vi "Update Mouse Move.vi"(8 "error in (no error)":errorcluster, 10 "Mouse Move":T1, 11 "Map Model in":refnum<class "Map Model.lvclass">) -> (0 "error out":errorcluster, 3 "Map Model out":refnum<class "Map Model.lvclass">)   [LabVIEW 2020, in "Map Model.lvlib" / "Map Model.lvclass"]
uses:
  Map Model.lvclass
  <vilib>/Utility/miscctls.llb/LVPoint32TypeDef.ctl
  Map Model.lvclass/Map Model.ctl
  Tools/Tool/Tool.lvclass
panel:
  # "NOTICE -- YOU MUST LEAVE THIS NOTICE IN PLACE.\n\nCopyright (c) 2017, LIANG LIU Shawn.Liu.cn@gmail.com\nAll rights reserved.\n\nRedistribution and use in source and binary forms, with or without modification, are permitted provided that the following conditions are met:\n-Redistributions of source code must retain the above copyright notice, this list of conditions and the following disclaimer.\n-Redistributions in binary form must reproduce the above copyright notice, this list of conditions and the following disclaimer in the documentation and/or other materials provided with the distribution.\n-Neither the name of the eLp nor the names of its contributors may be used to endorse or promote products derived from this software without specific prior written permission.\n\nTHIS SOFTWARE IS PROVIDED BY THE COPYRIGHT HOLDERS AND CONTRIBUTORS \"AS IS\" AND ANY EXPRESS OR IMPLIED WARRANTIES, INCLUDING, BUT NOT LIMITED TO, THE IMPLIED WARRANTIES OF MERCHANTABILITY AND FITNESS FOR A PARTICULAR PURPOSE ARE DISCLAIMED. IN NO EVENT SHALL THE COPYRIGHT HOLDER OR CONTRIBUTORS BE LIABLE FOR ANY DIRECT, INDIRECT, INCIDENTAL, SPECIAL, EXEMPLARY, OR CONSEQUENTIAL DAMAGES (INCLUDING, BUT NOT LIMITED TO, PROCUREMENT OF SUBSTITUTE GOODS OR SERVICES; LOSS OF USE, DATA, OR PROFITS; OR BUSINESS INTERRUPTION) HOWEVER CAUSED AND ON ANY THEORY OF LIABILITY, WHETHER IN CONTRACT, STRICT LIABILITY, OR TORT (INCLUDING NEGLIGENCE OR OTHERWISE) ARISING IN ANY WAY OUT OF THE USE OF THIS SOFTWARE, EVEN IF ADVISED OF THE POSSIBILITY OF SUCH DAMAGE."
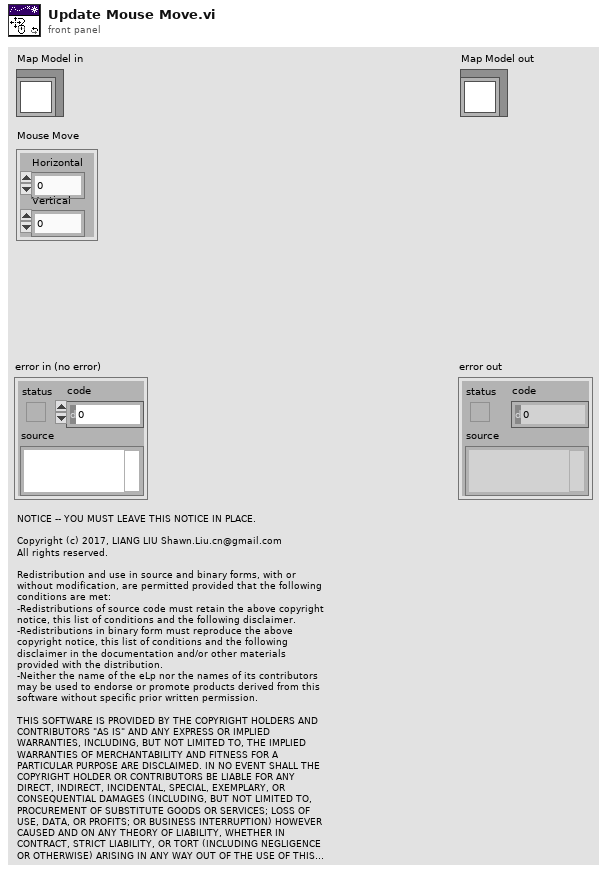
[diagram p1: front panel]
types:
  T1 = typedef "LVPoint32TypeDef.ctl" = cluster{"Horizontal":i32, "Vertical":i32}
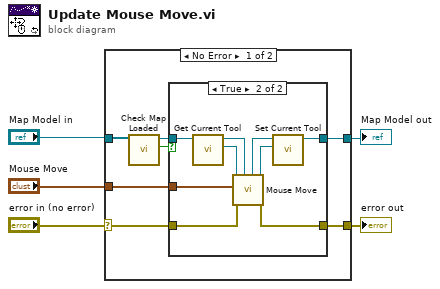
[diagram p0: block diagram]
diagram:
  n1 = case shown="No Error" "error in (no error)" {
    selector: "error in (no error)" -> [w6 w25]
    tunnel: "Map Model in" -> [w12 w24]
    tunnel: [w11 w24] -> w1
    tunnel: "Mouse Move" -> [w10 _]
    tunnel: [w9 w25] -> w2
    frame No Error {
      n2 = call "Check Map Loaded.vi"("Map Model in"=w12) -> ("Loaded"=w7:bool, "Map Model out"=w8:refnum<class "Map Model.lvclass">)  [unwired: 9 in]
      n3 = case shown="True" w7 {
        tunnel: [w14 w23] -> w11
        tunnel: w10 -> [_ w22]
        tunnel: [w13 w21] -> w9
        tunnel: w8 -> [w14 w18]
        tunnel: w6 -> [w13 w15]
        frame False {
        }
        frame True {
          n4 = call "Get Current Tool.vi"("Map Model in"=w18) -> ("Current Tool"=w17:refnum<class "Tool.lvclass">, "Map Model out"=w20:refnum<class "Map Model.lvclass">)  [unwired: 9 in]
          n5 = call-dynamic "Mouse Move.vi"("Map Model in"=w20, "error in (no error)"=w15, "Position"=w22, "Tool in"=w17) -> ("error out"=w21:errorcluster, "Tool out"=w16:refnum<class "Tool.lvclass">, "Map Model out"=w19:refnum<class "Map Model.lvclass">)  [unwired: 5 in]
          n6 = call "Set Current Tool.vi"("Current Tool"=w16, "Map Model in"=w19) -> ("Map Model out"=w23:refnum<class "Map Model.lvclass">)  [unwired: 9 in]
        }
      }
    }
    frame Error {
    }
  }
  "error out" <- w2
  "Map Model out" <- w1
